vi "API_Start Tool Module.vi"(8 "error in (no error)":errorcluster, 10 "Cfg File Path":path) -> (0 "error out":errorcluster, 1 "Wait for Event Sync?":bool, 2 "Tool Module Broadcast Events":T1)   [LabVIEW 2015, in "Tool Module.lvlib"]
doc: "Start the Tool Module Main.vi. The Cfg File Path is the path to the folder containing the Tool Configuration file (QC-X Tool Cfg.xml). The Tool Module will read this file in order to configure the tool unless the configuration comes from the tool's EEPROM. The file also contains the Operational Configuration data, where the two booleans 'Use Tool Cfg' and 'Use Tool Cal' determine whether the information from the file or from the tool is used.\n\nThis vi returns a cluster of events to be registered with the callers event structure. The callers event structure can then receive broadcast events generated by the Tool Module.\n\nCall the 'API_Wait on Module Start.vi' after registering the events provided by this vi to make sure that no Tool Module events are missed before the calling vi is ready to receive them."
uses:
  Tool Module.lvlib
  Broadcast Events--cluster.ctl
  Did Init Argument--cluster.ctl
  Status Updated Argument--cluster.ctl
  Error Reported Argument--cluster.ctl
  Stop Argument--cluster.ctl
  Get Module Execution Status Argument--cluster.ctl
  Send Status Argument--cluster.ctl
  Support/_STATUS Typedef--cluster.ctl
  Trigger Argument--cluster.ctl
  Connected Argument--cluster.ctl
  Read from File Rtn Argument--cluster.ctl
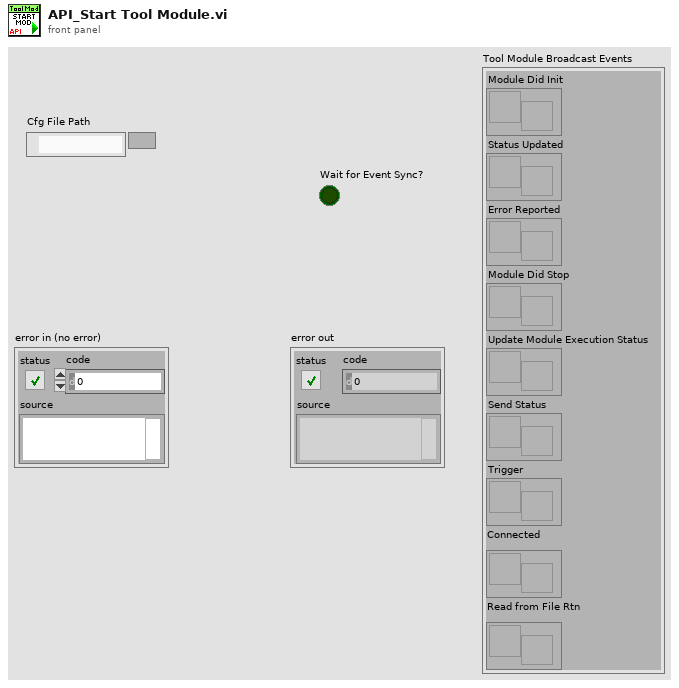
[diagram p1: front panel]
types:
  T1 = typedef "Tool Module.lvlib/Broadcast Events--cluster.ctl" = cluster{"Module Did Init":refnum<user-event>, "Status Updated":refnum<user-event>, "Error Reported":refnum<user-event>, "Module Did Stop":refnum<user-event>, "Update Module Execution Status":refnum<user-event>, "Send Status":refnum<user-event>, "Trigger":refnum<user-event>, "Connected":refnum<user-event>, "Read from File Rtn":refnum<user-event>}
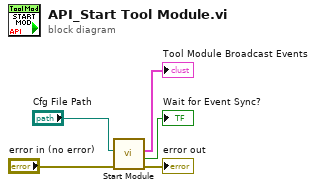
[diagram p0: block diagram]
diagram:
  n1 = call "Start Module.vi"("error in (no error)"="error in (no error)", "Cfg File Path"="Cfg File Path") -> ("error out"=→"error out":errorcluster, "Wait for Event Sync?"=→"Wait for Event Sync?":bool, "Tool Module Broadcast Events"=→"Tool Module Broadcast Events":T1)  [unwired: 7 in]
